vi "Bounds.vi"(1 "XRef":refnum<vi>, 2 "State In":T2) -> (0 "Bounds":cluster{"Width":T1, "Height":T1})   [LabVIEW 2018, in "ConPane Wrapper.xnode"]
uses:
  ConPane Wrapper.xnode
  State.ctl
  <vilib>/picture/picture.llb/imagedata.ctl
  <vilib>/XNodeSupport/XNodeTerm3Array.ctl
  <vilib>/XNodeSupport/XNodeTerm3.ctl
  <vilib>/XNodeSupport/XNodeString.ctl
  <vilib>/XNodeSupport/XNodeVariant.ctl
  <vilib>/XNodeSupport/XNodeRect32.ctl
  <vilib>/XNodeSupport/XNodeInt.ctl
  <vilib>/XNodeSupport/XNodeBool.ctl
  <vilib>/XNodeSupport/XNodeTermDirection.ctl
  Subvis/Term Types.ctl
  Subvis/Term Type.ctl
  <vilib>/XNodeSupport/NI_XNodeSupport.lvlib
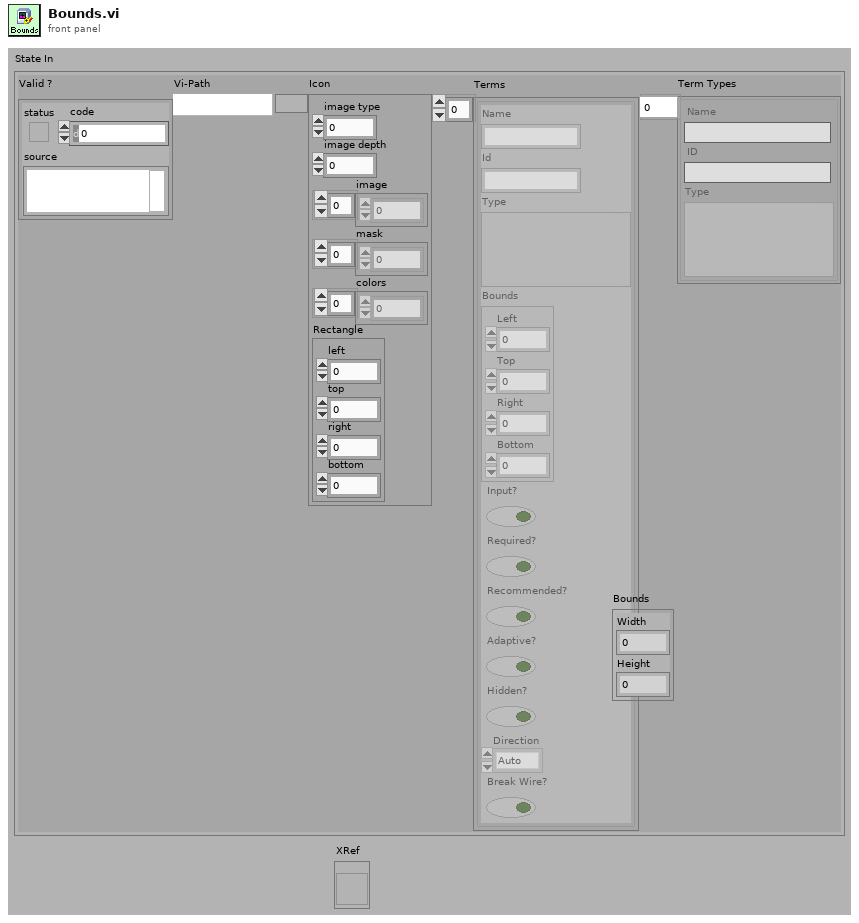
[diagram p1: front panel]
types:
  T1 = typedef "NI_XNodeSupport.lvlib/XNodeInt.ctl" = i32
  T2 = typedef "ConPane Wrapper.xnode/State.ctl" = cluster{"Valid ?":errorcluster, "Vi-Path":path, "Icon":T3, "Terms":T4, "Term Types":T11}
  T3 = typedef "imagedata.ctl" = cluster{"image type":i32, "image depth":i32, "image":u8[], "mask":u8[], "colors":u32[], "Rectangle":cluster{"left":i16, "top":i16, "right":i16, "bottom":i16}}
  T4 = typedef "NI_XNodeSupport.lvlib/XNodeTerm3Array.ctl" = T5[]
  T5 = typedef "NI_XNodeSupport.lvlib/XNodeTerm3.ctl" = cluster{"Name":T6, "Id":T6, "Type":T7, "Bounds":T8, "Input?":T9, "Required?":T9, "Recommended?":T9, "Adaptive?":T9, "Hidden?":T9, "Direction":T10, "Break Wire?":T9}
  T6 = typedef "NI_XNodeSupport.lvlib/XNodeString.ctl" = string
  T7 = typedef "NI_XNodeSupport.lvlib/XNodeVariant.ctl" = variant
  T8 = typedef "NI_XNodeSupport.lvlib/XNodeRect32.ctl" = cluster{"Left":T1, "Top":T1, "Right":T1, "Bottom":T1}
  T9 = typedef "NI_XNodeSupport.lvlib/XNodeBool.ctl" = bool
  T10 = typedef "NI_XNodeSupport.lvlib/XNodeTermDirection.ctl" = enum32{"Auto", "Up", "Down", "Left", "Right", "Center"}
  T11 = typedef "Term Types.ctl" = T12[]
  T12 = typedef "Term Type.ctl" = cluster{"Name":string, "ID":string, "Type":variant}
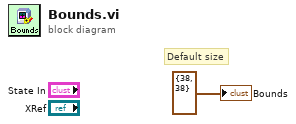
[diagram p0: block diagram]
diagram:
  # "Default size"
  "Bounds" <- cluster{"Width":T1, "Height":T1} {"Width"=38, "Height"=38} ("Bounds")
